vi "TestM1M3IRQPerformance.vi"() -> ()   [LabVIEW 2016]
uses:
  <vilib>/FPGAPlugInAG/Dynamic/niLvFpga_Close_Dynamic.vi
  <vilib>/Utility/error.llb/Error Cluster From Error Code.vi
  <vilib>/rvi/errors/niLvFpgaAdjustHostInterfaceError.vi
  <vilib>/RVI Host/nirviSupport.llb/nirviErrorClusterFromErrorCode.vi
  <vilib>/FPGAPlugInAG/Dynamic/niLvFpga_Run_Dynamic.vi
  <vilib>/FPGAPlugInAG/Dynamic/niLvFpga_Reset_Dynamic.vi
  <vilib>/FPGAPlugInAG/Dynamic/niLvFpga_Abort_Dynamic.vi
  <vilib>/rvi/interface/common/dynamic/niFpgaDynamicAddResources.vi
  <vilib>/FPGAPlugInAG/cRIO-9039 (Sync)/niLvFpga_Open_cRIO-9039 (Sync).vi
  <vilib>/rvi/interface/nirviCloseFPGA/nirviCloseFPGA.xnode
  <vilib>/rvi/interface/nirviMethod/nirviMethod.xnode
  <vilib>/rvi/interface/nirviOpenFPGA/nirviOpenFPGA.xnode
  FPGA Bitfiles/M1M3Support.lvbitx
  <vilib>/FPGAPlugInAG/Dynamic/niLvFpga_WriteFifo_Dynamic.vi
  <vilib>/rvi/errors/niLvFpgaMergeErrorWithErrorCode.vi
  <vilib>/rvi/interface/nirviMethod/StockFPGA_InlinedMethodWaitForMultipleIRQ.vi
  <vilib>/FPGAPlugInAG/Dynamic/niLvFpga_WaitOnIrq_Dynamic.vi
  <vilib>/FPGAPlugInAG/Dynamic/niLvFpga_AcknowledgeIrq_Dynamic.vi
panel:
  out "Iterations":i32
  out "Time (us)":u32
  in  "Boolean":bool
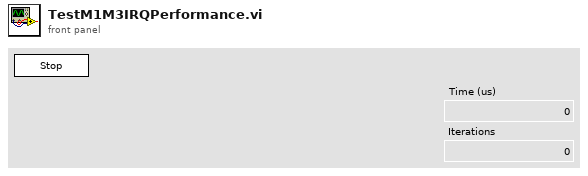
[diagram p1: front panel]
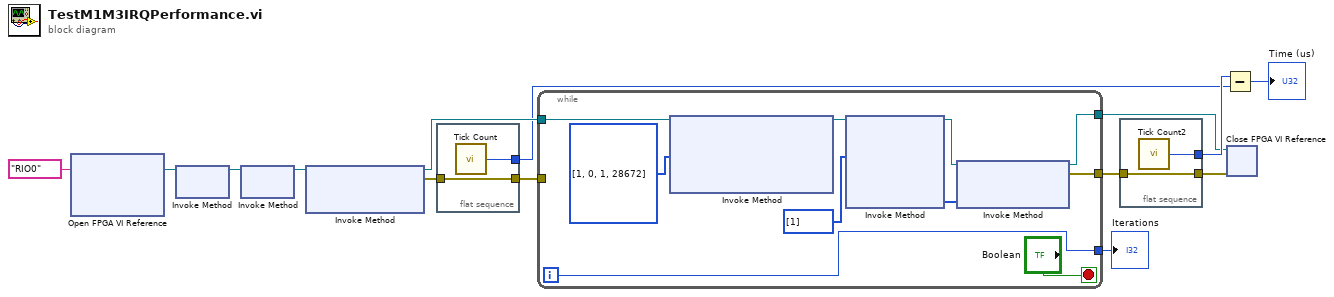
[diagram p0: block diagram]
diagram:
  n1 = xnode "Open FPGA VI Reference"("resource name"=tag "RIO0") -> ("FPGA VI Reference Out"=w14:refnum<k20>)  [unwired: 1 in, 1 out]
  n2 = xnode "Invoke Method"("FPGA VI Reference In"=w14) -> ("FPGA VI Reference Out"=w13:refnum<k20>)  [unwired: 1 in, 1 out]
  n3 = xnode "Invoke Method"("FPGA VI Reference In"=w13) -> ("FPGA VI Reference Out"=w12:refnum<k20>)  [unwired: 1 in, 1 out]
  n4 = xnode "Invoke Method"("FPGA VI Reference In"=w12) -> ("FPGA VI Reference Out"=w11:refnum<k20>, "error out"=w9:errorcluster)  [unwired: 2 in]
  n5 = flat-sequence {
    tunnel: [w16] -> w10
    tunnel: w9 -> [w16]
    tunnel: [w15] -> w6
    frame #0 {
      n6 = call "Tick Count"() -> ("Tick Count(uSec)"=w15:u32)
    }
  }
  n7 = while {
    tunnel: w11 -> [w26]
    tunnel: w10 -> [_]
    tunnel: [w19] -> w8
    tunnel: [w18] -> w4
    tunnel: [w17] -> w1
    i -> [w17]
    stop <- "Boolean" stop-if-true
    n8 = xnode "Invoke Method"("FPGA VI Reference In"=w26, "Data"=u16[] [1, 0, 1, 28672]) -> ("FPGA VI Reference Out"=w24:refnum<k20>)  [unwired: 2 in, 2 out]
    n9 = xnode "Invoke Method"("FPGA VI Reference In"=w24, "IRQ Number(s)"=i32[] [1]) -> ("FPGA VI Reference Out"=w22:refnum<k20>, "IRQ(s) Asserted"=w21:i32[])  [unwired: 2 in, 2 out]
    n10 = xnode "Invoke Method"("FPGA VI Reference In"=w22, "IRQ Number(s)"=w21) -> ("FPGA VI Reference Out"=w18:refnum<k20>, "error out"=w19:errorcluster)  [unwired: 1 in]
  }
  "Iterations" <- w1
  n11 = flat-sequence {
    tunnel: w8 -> [w27]
    tunnel: [w28] -> w7
    tunnel: [w27] -> w3
    frame #0 {
      n12 = call "Tick Count2"() -> ("Tick Count(uSec)"=w28:u32)
    }
  }
  n13 = Subtract(x=w7, y=w6) -> (x-y=→"Time (us)":u32)
  n14 = xnode "Close FPGA VI Reference"("FPGA VI Reference In"=w4, "error in"=w3) -> ()  [unwired: 1 out]
